vi "List Devices.vi"(8 "error in (no error)":errorcluster, 10 "Filter (Device Description)":string="Model 7008") -> (0 "error out":errorcluster, 2 "Devices":T1(array[cluster]))   [LabVIEW 2019, in "D2XX-lv.lvlib"]
uses:
  D2XX-lv.lvlib
  D2XX_Functions_7.0/FT_Open_Device_By_Serial_Number.vi
  private/FT_Status to Error.vi
  private/Open Device (serial number).vi
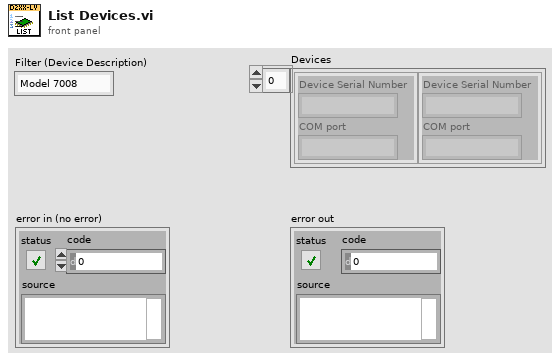
[diagram p1: front panel]
types:
  T1 = cluster{"Device Serial Number":string, "COM port":string}[]
  T2 = cluster{"Device Serial Number":string, "COM port":string}
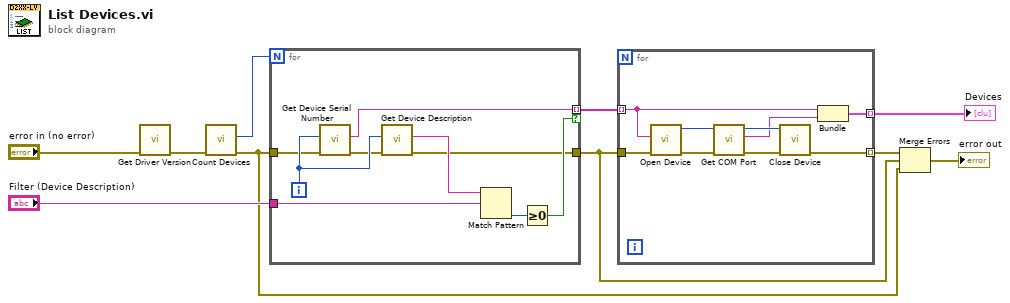
[diagram p0: block diagram]
diagram:
  n1 = call "Get Driver Version.vi"("error in (no error)"="error in (no error)") -> ("error out"=w6:errorcluster)  [unwired: 9 in, 1 out]
  n2 = call "Count Devices.vi"("error in (no error)"=w6) -> ("error out"=w1:errorcluster, "Number of Devices"=w4:i32)  [unwired: 9 in]
  n3 = for {
    N: w4 -> [_]
    tunnel: [w17] -> w5 mode=indexing if=w14
    tunnel: "Filter (Device Description)" -> [w13]
    tunnel: w1 -> [w12]
    tunnel: [w11] -> w2
    i -> [w19]
    n4 = call "Get Device Serial Number.vi"("error in (no error)"=w12, "Device Index"=w19) -> ("error out"=w18:errorcluster, "Device Serial Number"=w17:string)  [unwired: 8 in]
    n5 = call "Get Device Description.vi"("error in (no error)"=w18, "Device Index"=w19) -> ("error out"=w11:errorcluster, "Device Description"=w16:string)  [unwired: 8 in]
    n6 = Match Pattern(string=w16, regular expression=w13) -> (offset past match=w15:i32)  [unwired: 1 in, 3 out]
    n7 = Greater Or Equal To 0?(x=w15) -> (x >= 0?=w14:bool)
  }
  n8 = for {
    tunnel: w5 -> [w23] mode=indexing
    tunnel: w2 -> [w26]
    tunnel: [w21] -> w9 mode=indexing
    tunnel: [w20] -> w3 mode=indexing
    n9 = call-poly "Open Device.vi"("error in (no error)"=w26, "Device Serial Number"=w23) -> ("error out"=w25:errorcluster, "Handle"=w28:u32)  [unwired: 8 in]
    n10 = call "Get COM Port.vi"("error in (no error)"=w25, "Handle"=w28) -> ("error out"=w24:errorcluster, "COM port"=w22:string, "Handle out"=w27:u32)  [unwired: 7 in]
    n11 = call "Close Device.vi"("error in (no error)"=w24, "Handle"=w27) -> ("error out"=w20:errorcluster)  [unwired: 9 in]
    n12 = Bundle("Device Serial Number"=w23, "COM port"=w22) -> (w21:T2)  [unwired: 1 in]
  }
  "Devices" <- w9
  n13 = Merge Errors(w3, w2, w1) -> (→"error out":errorcluster)
